vi "get images.vi"(8 "error in (no error)":errorcluster, 11 "Room in":refnum<class "Room.lvclass">) -> (0 "error out":errorcluster, 2 "images":T1[](array[typedef]), 3 "Room out":refnum<class "Room.lvclass">)   [LabVIEW 2016, in "Room.lvclass"]
uses:
  Room.lvclass
  <vilib>/picture/picture.llb/imagedata.ctl
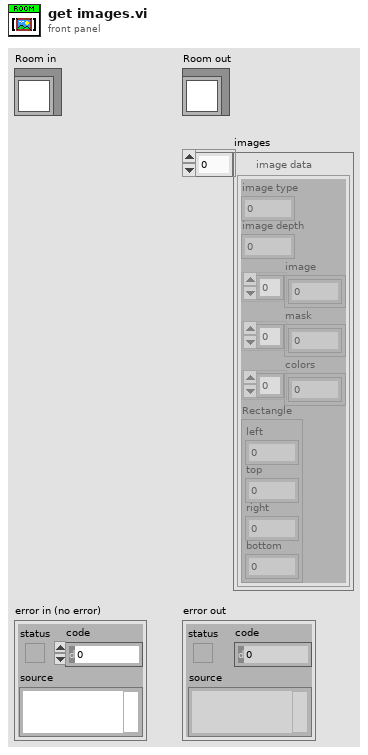
[diagram p1: front panel]
types:
  T1 = typedef "imagedata.ctl" = cluster{"image type":i32, "image depth":i32, "image":u8[], "mask":u8[], "colors":u32[], "Rectangle":cluster{"left":i16, "top":i16, "right":i16, "bottom":i16}}
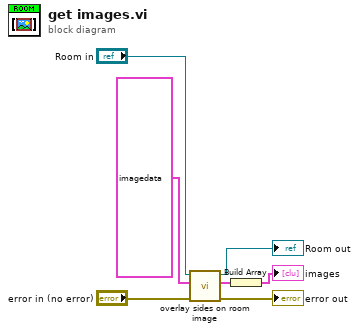
[diagram p0: block diagram]
diagram:
  n1 = call "overlay sides on room image.vi"("error in (no error)"="error in (no error)", "image data in"=T1 {"image type"=0, "image depth"=24, "image"=array[27648 elements], "mask"=[], "colors"=[], "Rectangle"={"left"=0, "top"=0, "right"=96, "bottom"=96}} ("image data"), "Room in"="Room in") -> ("error out"=→"error out":errorcluster, "image data  out"=w4:T1, "Room out"=→"Room out":refnum<class "Room.lvclass">)  [unwired: 6 in]
  n2 = Build Array(w4) -> (→"images":T1[])
